vi "CMD_EULER2QUAT.vi"(6 "Gantry in":refnum<class "Gantry.lvclass">, 8 "error in (no error)":errorcluster, 10 "Arguments":string[](array[string]), 11 "gScript Interpreter in":refnum<class "gScript Interpreter.lvclass">) -> (0 "error out":errorcluster, 3 "gScript Interpreter out":refnum<class "gScript Interpreter.lvclass">, 4 "Gantry out":refnum<class "Gantry.lvclass">)   [LabVIEW 2022 SP3, in "gScript Interpreter.lvclass"]
uses:
  gScript Interpreter.lvclass
  gScript Interpreter.lvclass/gScript Interpreter.ctl
  Shared Components/Orient3d Class/Orient3d.lvclass
  Shared Components/Gantry Class/Gantry.lvclass
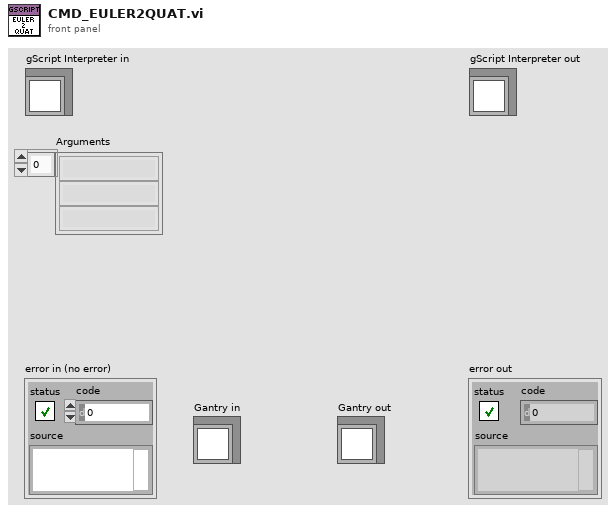
[diagram p1: front panel]
types:
  T1 = typedef "Memory Cell.ctl" = cluster{"type":T2, "x":dbl, "y":dbl, "z":dbl, "w":dbl}
  T2 = typedef "Memory Cell Type Enum.ctl" = enum16{"integer", "float", "vector", "rotation"}
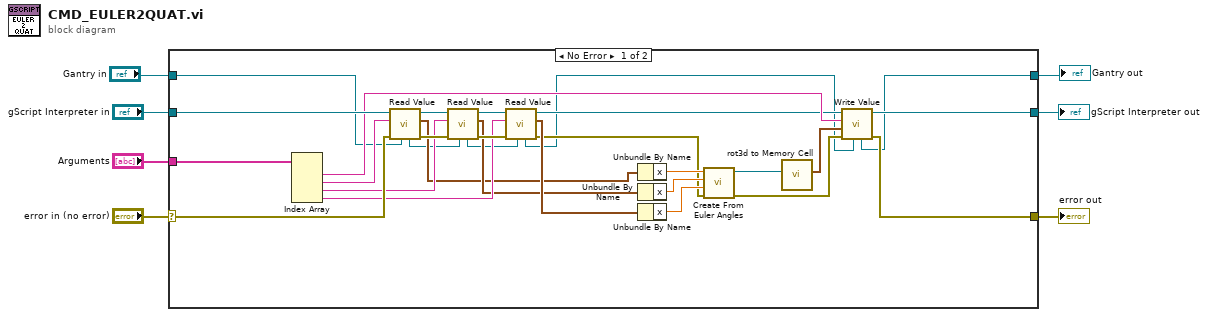
[diagram p0: block diagram]
diagram:
  n1 = case shown="No Error" "error in (no error)" {
    selector: "error in (no error)" -> [w34 w39]
    tunnel: [w27 w39] -> w6
    tunnel: [w28 w38] -> w4
    tunnel: "gScript Interpreter in" -> [w35 w38]
    tunnel: "Arguments" -> [w36 _]
    tunnel: "Gantry in" -> [w12 w37]
    tunnel: [w8 w37] -> w1
    frame No Error {
      n2 = Index Array(array=w36) -> (element #1=w29:string, element #2=w33:string, element #3=w30:string, element #4=w23:string)  [unwired: 4 in]
      n3 = call-dynamic "Read Value.vi"("Gantry in"=w12, "error in (no error)"=w34, "String in"=w33, "gScript Interpreter in"=w35) -> ("error out"=w32:errorcluster, "Memory Cell"=w20:T1, "gScript Interpreter out"=w31:refnum<class "gScript Interpreter.lvclass">, "Gantry out"=w11:refnum<class "Gantry.lvclass">)  [unwired: 4 in]
      n4 = call-dynamic "Read Value.vi"("Gantry in"=w11, "error in (no error)"=w32, "String in"=w30, "gScript Interpreter in"=w31) -> ("error out"=w24:errorcluster, "Memory Cell"=w21:T1, "gScript Interpreter out"=w25:refnum<class "gScript Interpreter.lvclass">, "Gantry out"=w10:refnum<class "Gantry.lvclass">)  [unwired: 4 in]
      n5 = call-dynamic "Read Value.vi"("Gantry in"=w10, "error in (no error)"=w24, "String in"=w23, "gScript Interpreter in"=w25) -> ("error out"=w16:errorcluster, "Memory Cell"=w22:T1, "gScript Interpreter out"=w15:refnum<class "gScript Interpreter.lvclass">, "Gantry out"=w9:refnum<class "Gantry.lvclass">)  [unwired: 4 in]
      n6 = Unbundle By Name(w20) -> ("x"=w19:dbl)
      n7 = Unbundle By Name(w21) -> ("x"=w18:dbl)
      n8 = Unbundle By Name(w22) -> ("x"=w17:dbl)
      n9 = call "Create From Euler Angles.vi"("error in"=w16, "phi/roll"=w17, "theta/pitch"=w18, "psi/yaw"=w19) -> ("error out"=w13:errorcluster, "Orient3d out"=w14:refnum<class "Orient3d.lvclass">)  [unwired: 6 in]
      n10 = call "rot3d to Memory Cell.vi"("Orient3d in"=w14) -> ("Memory Cell"=w26:T1)  [unwired: 10 in]
      n11 = call-dynamic "Write Value.vi"("Gantry in"=w9, "error in (no error)"=w13, "Value"=w26, "Address"=w29, "gScript Interpreter in"=w15) -> ("error out"=w27:errorcluster, "gScript Interpreter out"=w28:refnum<class "gScript Interpreter.lvclass">, "Gantry out"=w8:refnum<class "Gantry.lvclass">)  [unwired: 4 in]
    }
    frame Error {
    }
  }
  "error out" <- w6
  "gScript Interpreter out" <- w4
  "Gantry out" <- w1
